vi "Exec Command.vi"(0 "TCP In":refnum<k5>, 5 "Function Name":string, 9 "Timeout":i32=10, 11 "Error In":errorcluster) -> (4 "TCP Out":refnum<k5>, 6 "Return Value":string, 8 "OK Ack":string, 10 "Exception":string, 15 "Error Out":errorcluster)   [LabVIEW 2016, in "OPI.lvclass"]
uses:
  OPI.lvclass
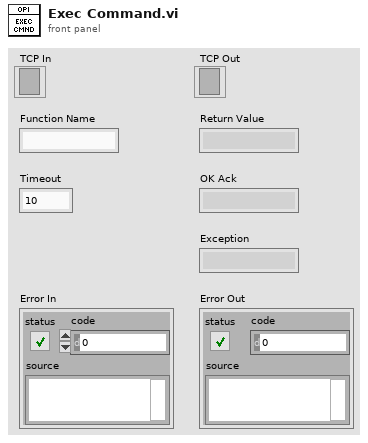
[diagram p1: front panel]
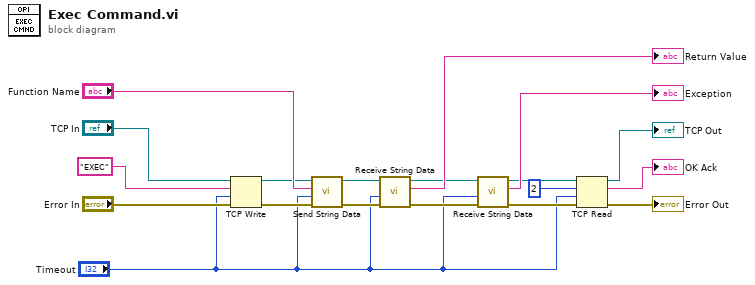
[diagram p0: block diagram]
diagram:
  n1 = TCP Write(connection ID="TCP In", data in="EXEC", error in (no error)="Error In", 9:"Timeout") -> (connection ID out=w7:refnum<k5>, error out=w6:errorcluster)  [unwired: 1 out]
  n2 = call "Send String Data.vi"("Error In"=w6, "timeout ms (25000)"="Timeout", "String Data"="Function Name", "TCP In"=w7) -> ("Error Out"=w16:errorcluster, "TCP Out"=w14:refnum<k5>)  [unwired: 6 in]
  n3 = call "Receive String Data.vi"("Error In"=w16, "timeout ms (25000)"="Timeout", "TCP In"=w14) -> ("Error Out"=w19:errorcluster, "String Data"=→"Return Value":string, "TCP Out"=w15:refnum<k5>)  [unwired: 6 in]
  n4 = call "Receive String Data.vi"("Error In"=w19, "timeout ms (25000)"="Timeout", "TCP In"=w15) -> ("Error Out"=w4:errorcluster, "String Data"=→"Exception":string, "TCP Out"=w5:refnum<k5>)  [unwired: 6 in]
  n5 = TCP Read(connection ID=w5, bytes to read=2, error in (no error)=w4, 9:"Timeout") -> (connection ID out=→"TCP Out":refnum<k5>, data out=→"OK Ack":string, error out=→"Error Out":errorcluster)  [unwired: 1 in]
